vi "UI.SerialCode.vi"(7 "Last SN":string, 9 "条码长度":i32=13, 10 "预制信息":string, 11 "AutoClose?":bool) -> (1 "Serial Number":string, 3 "OK?":bool)   [LabVIEW 2012, in "Lib_UEL.ATE.lvlib" / "Lib_App.lvlib"]
uses:
  Lib_App.lvlib
panel:
  out "Mode:":enum16{"Serial Number"}(ring)
  in  "Cancel":bool
  in  "OK":bool
  in  "Code:":string
  # "V 1.0 初始版本.\nV 1.1 增加快捷键L, 会自动输入上次条码, 或者'0...'"
  # "字母键'L'会自动输入上次扫描的条码."
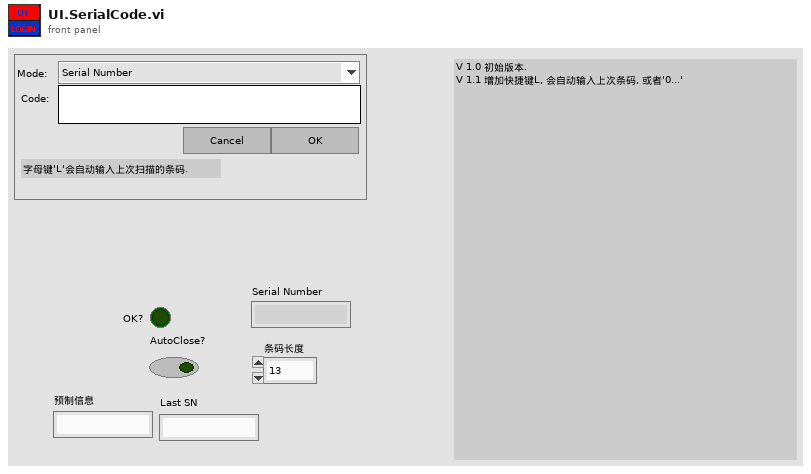
[diagram p1: front panel]
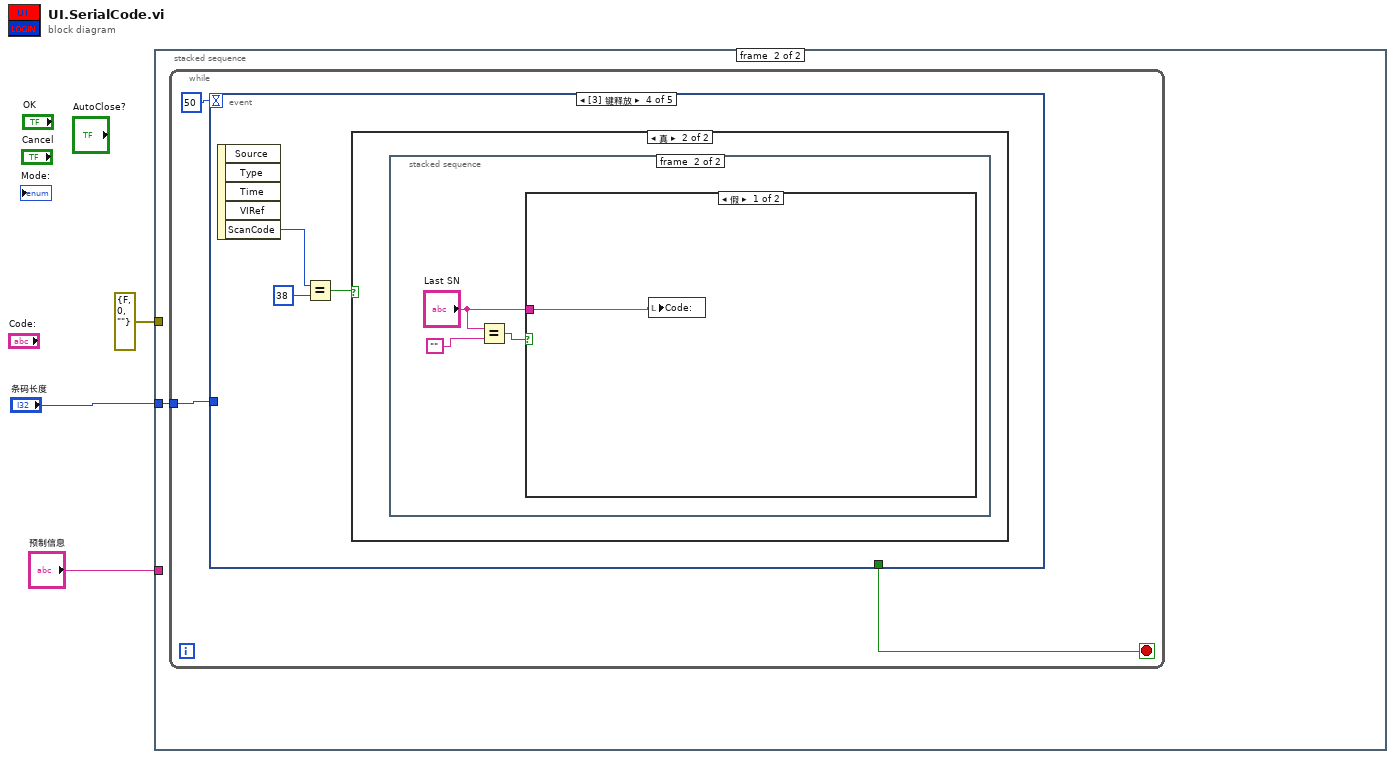
[diagram p0: block diagram]
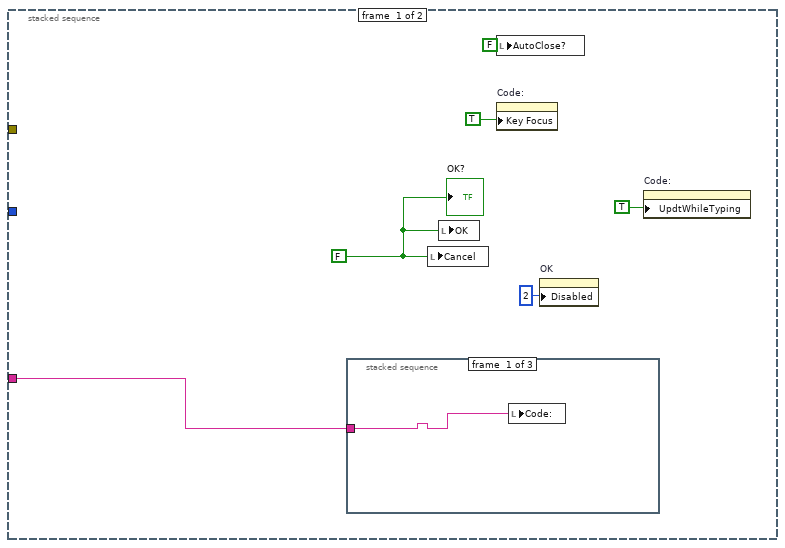
[diagram p2: hidden frame]
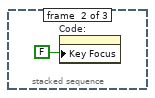
[diagram p3: hidden frame]
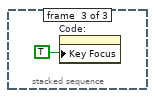
[diagram p4: hidden frame]
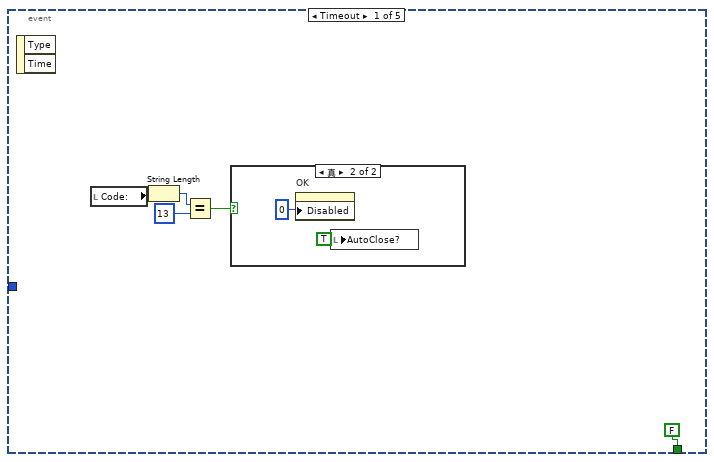
[diagram p5: hidden frame]
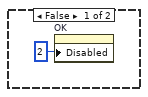
[diagram p6: hidden frame]
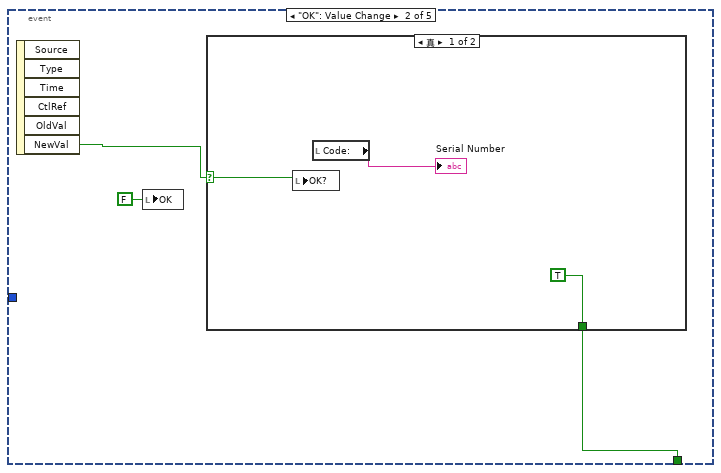
[diagram p7: hidden frame]
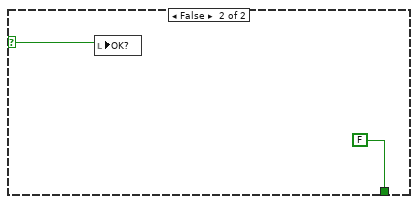
[diagram p8: hidden frame]
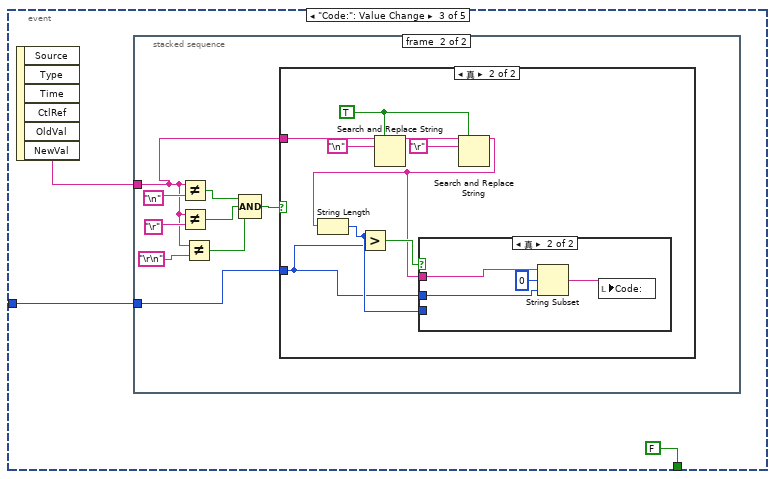
[diagram p9: hidden frame]
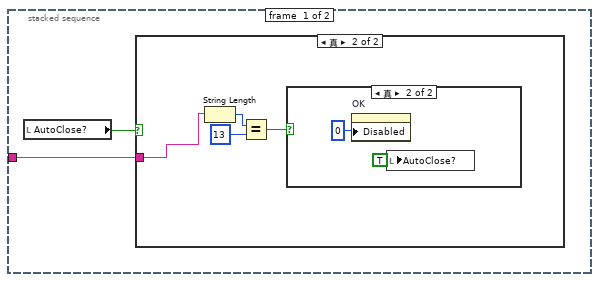
[diagram p10: hidden frame]
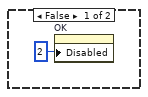
[diagram p12: hidden frame]
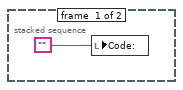
[diagram p16: hidden frame]
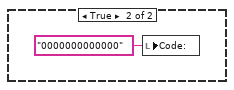
[diagram p17: hidden frame]
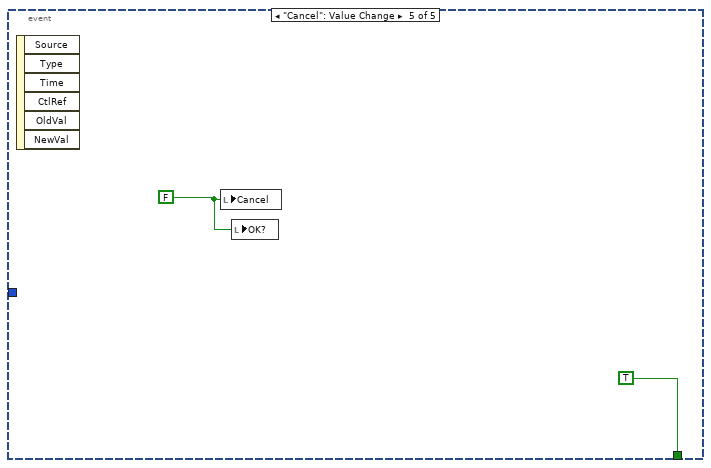
[diagram p18: hidden frame]
diagram:
  n1 = stacked-sequence {
    tunnel: errorcluster {"status"=FALSE, "code"=0, "source"=""} ("error in (no error)") -> [_ _]
    tunnel: "条码长度" -> [_ w13]
    tunnel: "预制信息" -> [w4 _]
    frame #0 {
      w6 = FALSE ("Cancel")
      n2 = stacked-sequence {
        tunnel: w4 -> [w10 _ _]
        frame #0 {
          n3 = local write "Code:"(w10) -> ()
        }
        frame #1 {
          n4 = property on="Code:" class="Str"("Key Focus"=FALSE ("键选中")) -> ()  [unwired: 2 in, 2 out]
        }
        frame #2 {
          n5 = property on="Code:" class="Str"("Key Focus"=TRUE ("键选中")) -> ()  [unwired: 2 in, 2 out]
        }
      }
      n6 = local write "Cancel"(w6) -> ()
      n7 = local write "OK"(w6) -> ()
      n8 = local write "AutoClose?"(FALSE ("again?")) -> ()
      n9 = property on="Code:" class="Str"("Key Focus"=TRUE ("键选中")) -> ()  [unwired: 2 in, 2 out]
      n10 = property on="OK" class="Bool (严格)"("Disabled"=u8 2 ("禁用")) -> ()  [unwired: 2 in, 2 out]
      n11 = property on="Code:" class="Str"("UpdtWhileTyping"=TRUE ("键入时刷新？")) -> ()  [unwired: 2 in, 2 out]
      "OK?" <- w6
    }
    frame #1 {
      n12 = while {
        tunnel: w13 -> [w14]
        stop <- w15 stop-if-true
        n13 = event shown="[3] 键释放" {
          selector: _ -> [_ _ _ _ _]
          dyn-events: _ -> [_ _ _ _ _]
          timeout: 50 -> [_ _ _ _ _]
          tunnel: [FALSE w26 FALSE _ TRUE ("OK")] -> w15
          tunnel: w14 -> [_ _ w33 _ _]
          event Timeout {
            n14 = event-data() -> ()  [unwired: 1 in, 2 out]
            n15 = local read "Code:"() -> (w17:string)
            n16 = String Length(string=w17) -> (length=w19:i32)
            n17 = Equal?(x=w19, y=13) -> (x = y?=w20:bool)
            n18 = case shown="真" w20 {
              frame False {
                n19 = property on="OK" class="Bool (严格)"("Disabled"=u8 2 ("禁用")) -> ()  [unwired: 2 in, 2 out]
              }
              frame True {
                n20 = property on="OK" class="Bool (严格)"("Disabled"=u8 0 ("禁用")) -> ()  [unwired: 2 in, 2 out]
                n21 = local write "AutoClose?"(TRUE ("again?")) -> ()
              }
            }
          }
          event "OK": Value Change {
            n22 = event-data() -> ("NewVal"=w27:bool)  [unwired: 1 in, 5 out]
            n23 = local write "OK"(FALSE ("OK")) -> ()
            n24 = case shown="真" w27 {
              selector: w27 -> [w30 w32]
              tunnel: [TRUE FALSE] -> w26
              frame True {
                n25 = local write "OK?"(w30) -> ()
                n26 = local read "Code:"() -> (→"Serial Number":string)
              }
              frame False {
                n27 = local write "OK?"(w32) -> ()
              }
            }
          }
          event "Code:": Value Change {
            n28 = event-data() -> ("NewVal"=w34:string)  [unwired: 1 in, 5 out]
            n29 = stacked-sequence {
              tunnel: w34 -> [w36 w50]
              tunnel: w33 -> [_ w45]
              frame #0 {
                n30 = local read "AutoClose?"() -> (w37:bool)
                n31 = case shown="真" w37 {
                  tunnel: w36 -> [_ w38]
                  frame False {
                  }
                  frame True {
                    n32 = String Length(string=w38) -> (length=w40:i32)
                    n33 = Equal?(x=w40, y=13) -> (x = y?=w41:bool)
                    n34 = case shown="真" w41 {
                      frame False {
                        n35 = property on="OK" class="Bool (严格)"("Disabled"=u8 2 ("禁用")) -> ()  [unwired: 2 in, 2 out]
                      }
                      frame True {
                        n36 = property on="OK" class="Bool (严格)"("Disabled"=u8 0 ("禁用")) -> ()  [unwired: 2 in, 2 out]
                        n37 = local write "AutoClose?"(TRUE ("again?")) -> ()
                      }
                    }
                  }
                }
              }
              frame #1 {
                n38 = Not Equal?(x=w50, y="\n") -> (x != y?=w48:bool)
                n39 = Not Equal?(x=w50, y="\r") -> (x != y?=w47:bool)
                n40 = Not Equal?(x=w50, y="\r\n") -> (x != y?=w46:bool)
                n41 = Compound Arithmetic op=AND(w48, w47, w46) -> (w49:bool)
                n42 = case shown="真" w49 {
                  tunnel: w50 -> [_ w55]
                  tunnel: w45 -> [_ w54]
                  frame False {
                  }
                  frame True {
                    w60 = TRUE ("替换全部？(F)")
                    n43 = Search and Replace String(replace all?=w60, input string=w55, search string="\n") -> (result string=w61:string)  [unwired: 5 in, 3 out]
                    n44 = Search and Replace String(replace all?=w60, input string=w61, search string="\r") -> (result string=w56:string)  [unwired: 5 in, 3 out]
                    n45 = String Length(string=w56) -> (length=w57:i32)
                    n46 = Greater?(x=w57, y=w54) -> (0:w58:bool)
                    n47 = case shown="真" w58 {
                      tunnel: w56 -> [_ w66]
                      tunnel: w57 -> [_ _]
                      tunnel: w54 -> [_ w63]
                      frame False {
                      }
                      frame True {
                        n48 = String Subset(string=w66, offset (0)=0 ("偏移量(0)"), length (rest)=w63) -> (substring=w65:string)
                        n49 = local write "Code:"(w65) -> ()
                      }
                    }
                  }
                }
              }
            }
          }
          event Key Up {
            n50 = event-data() -> ("ScanCode"=w69:i16)  [unwired: 1 in, 4 out]
            n51 = Equal?(x=w69, y=i16 38) -> (x = y?=w67:bool)
            n52 = case shown="真" w67 {
              frame False {
              }
              frame True {
                n53 = stacked-sequence {
                  frame #0 {
                    n54 = local write "Code:"("") -> ()
                  }
                  frame #1 {
                    n55 = Equal?(x="Last SN", y="") -> (x = y?=w72:bool)
                    n56 = case shown="假" w72 {
                      tunnel: "Last SN" -> [w74 _]
                      frame False {
                        n57 = local write "Code:"(w74) -> ()
                      }
                      frame True {
                        n58 = local write "Code:"("0000000000000" ("Code:")) -> ()
                      }
                    }
                  }
                }
              }
            }
          }
          event "Cancel": Value Change {
            w77 = FALSE ("OK")
            n59 = event-data() -> ()  [unwired: 1 in, 6 out]
            n60 = local write "Cancel"(w77) -> ()
            n61 = local write "OK?"(w77) -> ()
          }
        }
      }
    }
  }
